vi "Ballard - Arinc-429 - Add Data Channel.vi"(8 "error in (no error)":errorcluster, 11 "Node Ptr":u64 format="%.0x") -> (0 "error out":errorcluster)   [LabVIEW 2017, in "Ballard Arinc-429 System Explorer.lvlib"]
uses:
  Ballard Arinc-429 System Explorer.lvlib
  <vilib>/NI Veristand/Custom Device API/Custom Device Channel.ctl
  <vilib>/NI Veristand/Custom Device API/Custom Device Channel Type.ctl
  Shared/Controls and Global/Global.vi
  <vilib>/NI Veristand/Custom Device API/Get Item Property (U32).vi
  RT Driver/SubVIs/ReadWrite/Extract BCD Parameter.vi
  Shared/Ballard Arinc-429 Shared.lvlib
  <vilib>/NI Veristand/Custom Device API/Custom Device API.lvlib
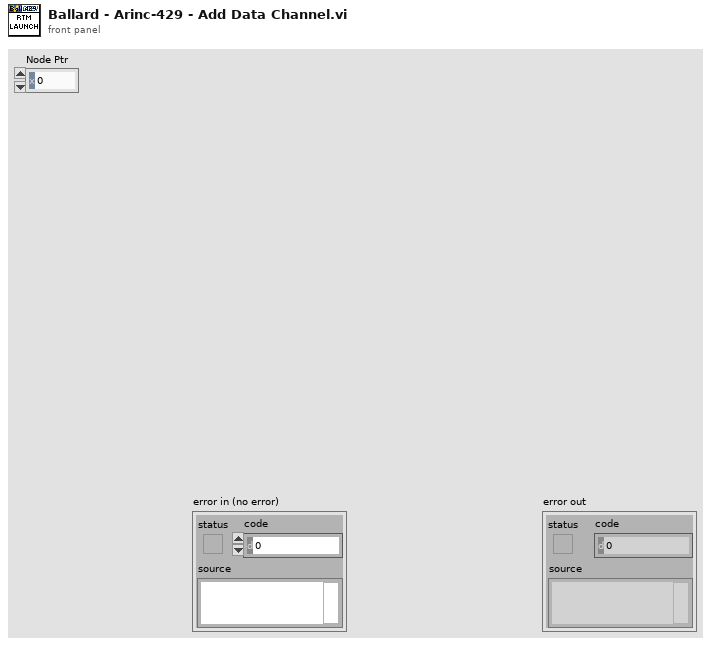
[diagram p1: front panel]
types:
  T1 = typedef "Custom Device API.lvlib/Custom Device Channel Type.ctl" = enum16{"Input", "Output"}
  T2 = typedef "Custom Device API.lvlib/Custom Device Channel.ctl" = cluster{"Type":T1, "Units":string, "Default Value":dbl, "Faultable":bool, "Scalable":bool}
  T3 = typedef "Custom Device API.lvlib/Custom Device Item Ref.ctl" = u64
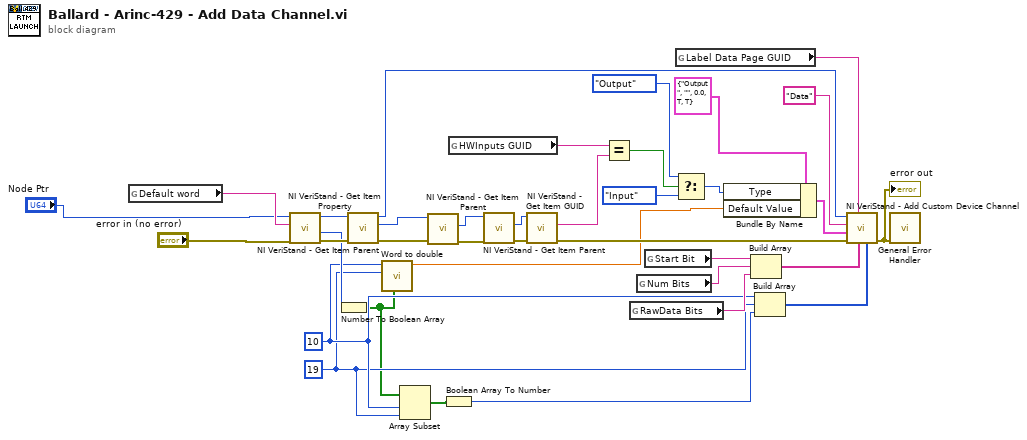
[diagram p0: block diagram]
diagram:
  w4 = 19
  w5 = 10
  n1 = global read "Global.vi" "Default word"() -> (w14:string)
  n2 = call-poly <vilib>:"NI VeriStand - Get Item Property.vi"("error in (no error)"="error in (no error)", "Property Name"=w14, "Item Ref in"="Node Ptr") -> ("error out"=w15:errorcluster, "Value"=w7:u32, "Item Ref out"=w16:T3)  [unwired: 5 in, 1 out]
  n3 = Number To Boolean Array(number=w7) -> (Boolean array=w1:bool[])
  n4 = call <vilib>:"NI VeriStand - Get Item Parent.vi"("error in (no error)"=w15, "Item Ref in"=w16) -> ("error out"=w9:errorcluster, "Parent Ref"=w11:T3, "Item Ref out"=w26:T3)  [unwired: 6 in, 1 out]
  n5 = call "Word to double.vi"("Word"=w1, "Number of Bits"=w4, "Start Bit"=w5) -> ("Double"=w17:dbl)  [unwired: 8 in]
  n6 = Array Subset(array=w1, index=w5, length=w4) -> (w3:bool[])
  n7 = call <vilib>:"NI VeriStand - Get Item Parent.vi"("error in (no error)"=w9, "Item Ref in"=w11) -> ("error out"=w8:errorcluster, "Parent Ref"=w10:T3)  [unwired: 6 in, 2 out]
  n8 = Boolean Array To Number(Boolean array=w3) -> (number=w2:u32)
  n9 = global read "Global.vi" "HWInputs GUID"() -> (w28:string)
  n10 = call <vilib>:"NI VeriStand - Get Item Parent.vi"("error in (no error)"=w8, "Item Ref in"=w10) -> ("error out"=w34:errorcluster, "Parent Ref"=w33:T3)  [unwired: 6 in, 2 out]
  n11 = call <vilib>:"NI VeriStand - Get Item GUID.vi"("error in (no error)"=w34, "Item Ref in"=w33) -> ("error out"=w21:errorcluster, "GUID"=w27:string)  [unwired: 7 in, 1 out]
  n12 = Equal?(x=w28, y=w27) -> (x = y?=w23:bool)
  n13 = global read "Global.vi" "RawData Bits"() -> (w6:string)
  n14 = global read "Global.vi" "Num Bits"() -> (w36:string)
  n15 = global read "Global.vi" "Start Bit"() -> (w24:string)
  n16 = global read "Global.vi" "Label Data Page GUID"() -> (w35:string)
  n17 = Select(t=Custom_Device_Channel_Type."Output" ("Type"), s=w23, f=Custom_Device_Channel_Type."Input" ("Type")) -> (s? t:f=w31:T1)
  n18 = Bundle By Name(cluster=T2 {"Type"=enum."Output", "Units"="", "Default Value"=0.0, "Faultable"=TRUE, "Scalable"=TRUE} ("Channel"), "Type"=w31, "Default Value"=w17) -> (w19:T2)
  n19 = Build Array(w24, w36, w6) -> (w25:string[])
  n20 = Build Array(w5, w4, w2) -> (w20:u32[])
  n21 = call <vilib>:"NI VeriStand - Add Custom Device Channel.vi"("Property Values"=w20, "Property names"=w25, "GUID (Default Channel)"=w35, "error in (no error)"=w21, "Channel"=w19, "Channel Name"="Data", "Parent Ref in"=w26) -> ("error out"=w22:errorcluster)  [unwired: 1 in, 3 out]
  "error out" <- w22
  n22 = call <vilib>:"General Error Handler.vi"("error in (no error)"=w22) -> ()  [unwired: 10 in, 5 out]
